vi "Get Axis Motion Status Motor Modified.vi"(8 "error in (no error)":errorcluster, 9 "Axis (1)":i32=1 min=1 max=3, 10 "VISA resource name":refnum<visa-resource-name>, 11 "ESP302 in":refnum<class "ESP302.lvclass">) -> (0 "error out":errorcluster, 1 "Motion Done":bool, 2 "VISA resource name out":refnum<visa-resource-name>, 3 "ESP302 out":refnum<class "ESP302.lvclass">)   [LabVIEW 2020, in "ESP302.lvclass"]
uses:
  ESP302/ESP302.lvclass
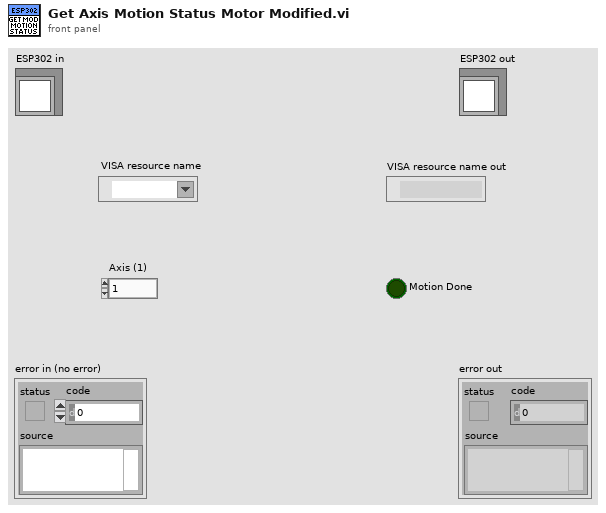
[diagram p1: front panel]
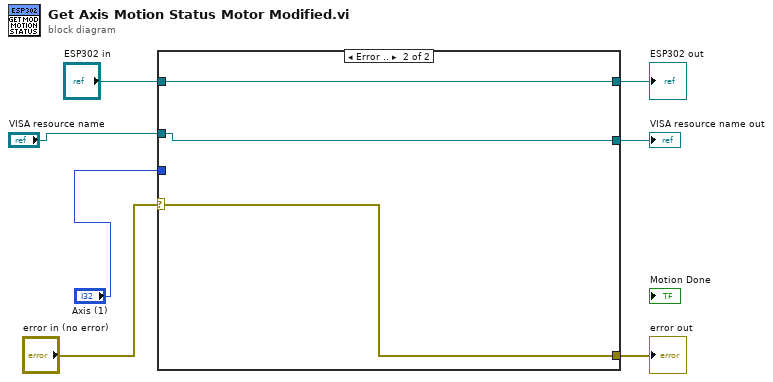
[diagram p0: block diagram]
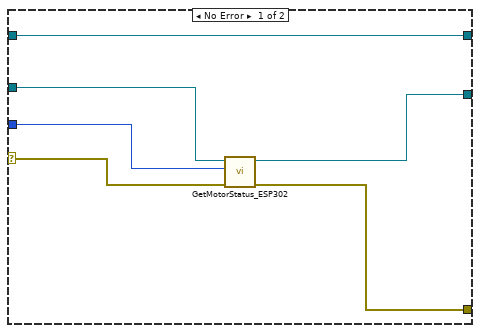
[diagram p2: hidden frame]
diagram:
  n1 = case shown="Error .." "error in (no error)" {
    selector: "error in (no error)" -> [w11 w14]
    tunnel: "ESP302 in" -> [w13 w16]
    tunnel: [w13 w16] -> w5
    tunnel: "VISA resource name" -> [w12 w15]
    tunnel: "Axis (1)" -> [w10 _]
    tunnel: [w9 w15] -> w2
    tunnel: [w8 w14] -> w1
    frame No Error {
      n2 = call "GetMotorStatus_ESP302.vi"("error in (no error)"=w11, "Axis (1)"=w10, "VISA resource name"=w12) -> ("error out"=w8:errorcluster, "VISA resource name out"=w9:refnum<visa-resource-name>)  [unwired: 3 in]
    }
    frame Error {
    }
  }
  "error out" <- w1
  "ESP302 out" <- w5
  "VISA resource name out" <- w2
